vi "setConfigDir.vi"(8 "error in (no error)":errorcluster, 10 "Config Dir":path=path "/home/ttsai/Documents/stash/ts_tcs_ofc/configData", 11 "OptStateEsti in":refnum<class "OptStateEsti.lvclass">) -> (0 "error out":errorcluster, 3 "OptStateEsti out":refnum<class "OptStateEsti.lvclass">)   [LabVIEW 2016, in "OptStateEsti.lvclass"]
doc: "Set the configuration directory."
uses:
  OptStateEsti.lvclass
  OptStateEsti.lvclass/OptStateEsti.ctl
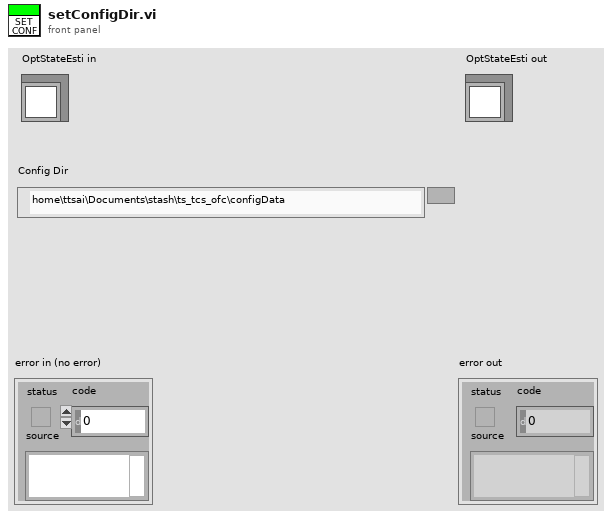
[diagram p1: front panel]
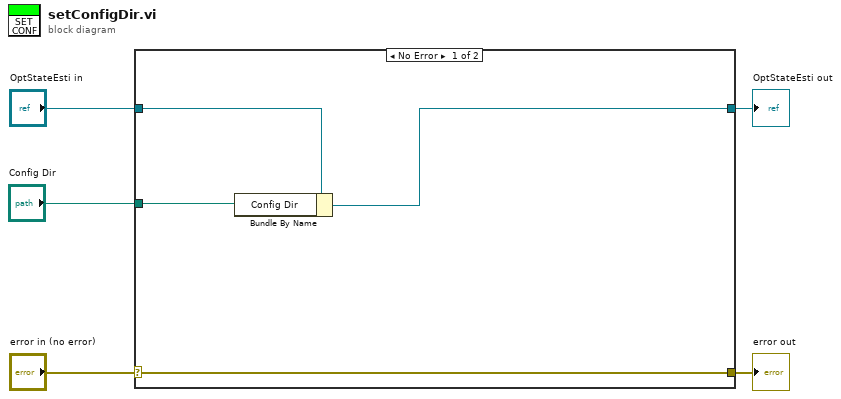
[diagram p0: block diagram]
diagram:
  n1 = case shown="No Error" "error in (no error)" {
    selector: "error in (no error)" -> [w9 w11]
    tunnel: [w9 w11] -> w4
    tunnel: [w6 w10] -> w2
    tunnel: "OptStateEsti in" -> [w8 w10]
    tunnel: "Config Dir" -> [w7 _]
    frame No Error {
      n2 = Bundle By Name(cluster=w8, "Config Dir"=w7) -> (w6:refnum<class "OptStateEsti.lvclass">)
    }
    frame Error {
    }
  }
  "error out" <- w4
  "OptStateEsti out" <- w2
